vi "Generate Unique Header.vi"(8 "error in":errorcluster, 11 "SOAP Data in":refnum<class "SOAP Data.lvclass">) -> (0 "error out":errorcluster, 2 "Header":string[](array[string]), 3 "SOAP Data out":refnum<class "SOAP Data.lvclass">)   [LabVIEW 2016, in "Controller.lvlib" / "SOAP Data.lvclass"]
uses:
  SOAP Data.lvclass
  <vilib>/MSR Consulting, LLC/General Reuse/Data/Data.lvclass
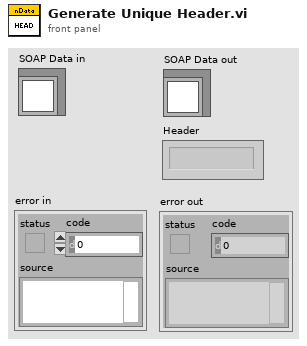
[diagram p1: front panel]
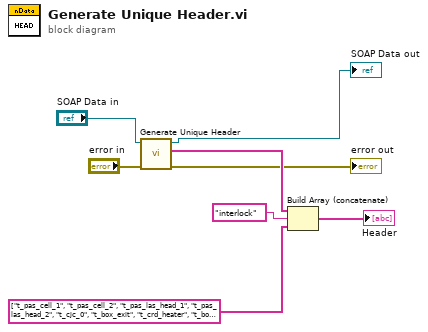
[diagram p0: block diagram]
diagram:
  n1 = call-parent "Generate Unique Header.vi"("error in"="error in", "Data in"="SOAP Data in") -> ("error out"=→"error out":errorcluster, "Header"=w5:string[], "Data out"=→"SOAP Data out":refnum<class "SOAP Data.lvclass">)  [unwired: 7 in]
  n2 = Build Array (concatenate)(w5, "interlock", string[] ["t_pas_cell_1", "t_pas_cell_2", "t_pas_las_head_1", "t_pas_las_head_2", "t_cjc_0", "t_box_exit", "t_crd_heater", "t_box_inlet", "t_crd_laser_head", "t_cjc_1"] ("Header")) -> (→"Header":string[])
